vi "Read CustomCanon.vi"(8 "error in (no error)":errorcluster, 11 "Canon in":refnum<class "Canon.lvclass">) -> (0 "error out":errorcluster, 2 "CustomCanon":string, 3 "Canon out":refnum<class "Canon.lvclass">)   [LabVIEW 2021, in "Canon.lvclass"]
uses:
  Canon.lvclass
  Canon.lvclass/Canon.ctl
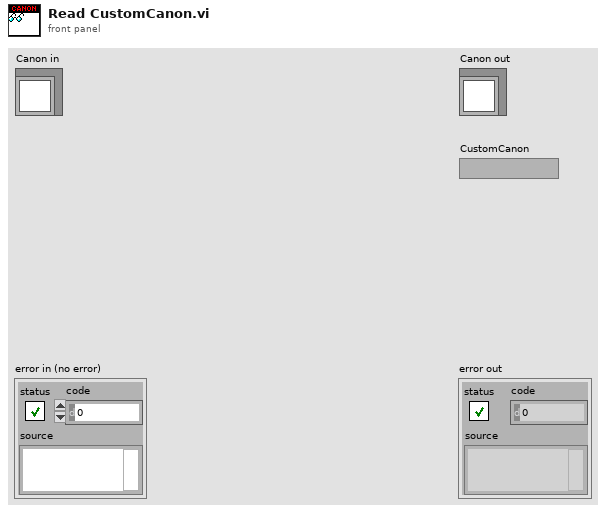
[diagram p1: front panel]
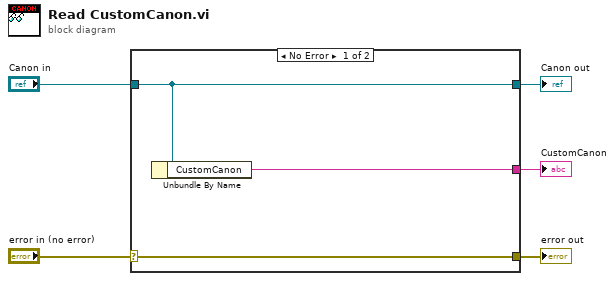
[diagram p0: block diagram]
diagram:
  n1 = case shown="No Error" "error in (no error)" {
    selector: "error in (no error)" -> [w8 w9]
    tunnel: [w8 w9] -> w4
    tunnel: [w7 w10] -> w2
    tunnel: "Canon in" -> [w7 w10]
    tunnel: [w6 _] -> w1
    frame No Error {
      n2 = Unbundle By Name(w7) -> ("CustomCanon"=w6:string)
    }
    frame Error {
    }
  }
  "error out" <- w4
  "Canon out" <- w2
  "CustomCanon" <- w1
